vi "Browse for XNET Database.vi"(8 "error in (no error)":errorcluster) -> (0 "error out":errorcluster, 1 "Cancel Out":bool, 2 "Import Path out":path, 3 "XNET Settings":T1={"Database"="", "Cluster"="", "Port"="", "Baud rate [Bd]"=0, "Termination"=0, "CAN I/O Mode"=0, "FD Baud rate [Bd]"=500000, "Priority"=100, "Use Legacy"=FALSE, "FD ISO Mode"=0, "Default Max Counter Value"=0.0, "Default Protect Type"=enum."Arb ID + Bytes Checksum with Inversion"} {"FD ISO Mode" items=["ISO", "Non ISO", "ISO Legacy"]; "CAN I/O Mode" items=["CAN 2.0", "CAN FD", "CAN FD+BRS"]; "Termination" items=["Off", "On"]})   [LabVIEW 2025, in "Protection and Counter Addon System Explorer.lvlib"]
uses:
  Protection and Counter Addon System Explorer.lvlib
  Addon Shared/Types/XNET Settings.ctl
  SubModules/Frame-Protection-Support/Source/Shared/Types/Protection Type.ctl
  <resource>/objmgr/xnet.rc
  Addon Shared/Protection and Counter Addon Shared.lvlib
  SubModules/Frame-Protection-Support/Source/Shared/Protection and Counter Support Shared.lvlib
panel:
  in  "Path":path caption="Previous Personality Path (Optional)"
  in  "FD Baud rate [Bd]":u64=500000
  out "CAN I/O Mode":u32(ring) items=["CAN 2.0", "CAN FD", "CAN FD+BRS"]
  in  "Baud rate [Bd]":u64=500000
  in  "Select CAN Cluster":u16(ring)
  in  "Cancel":bool
  in  "Select":bool
  in  "XNET Database":refnum<k21>
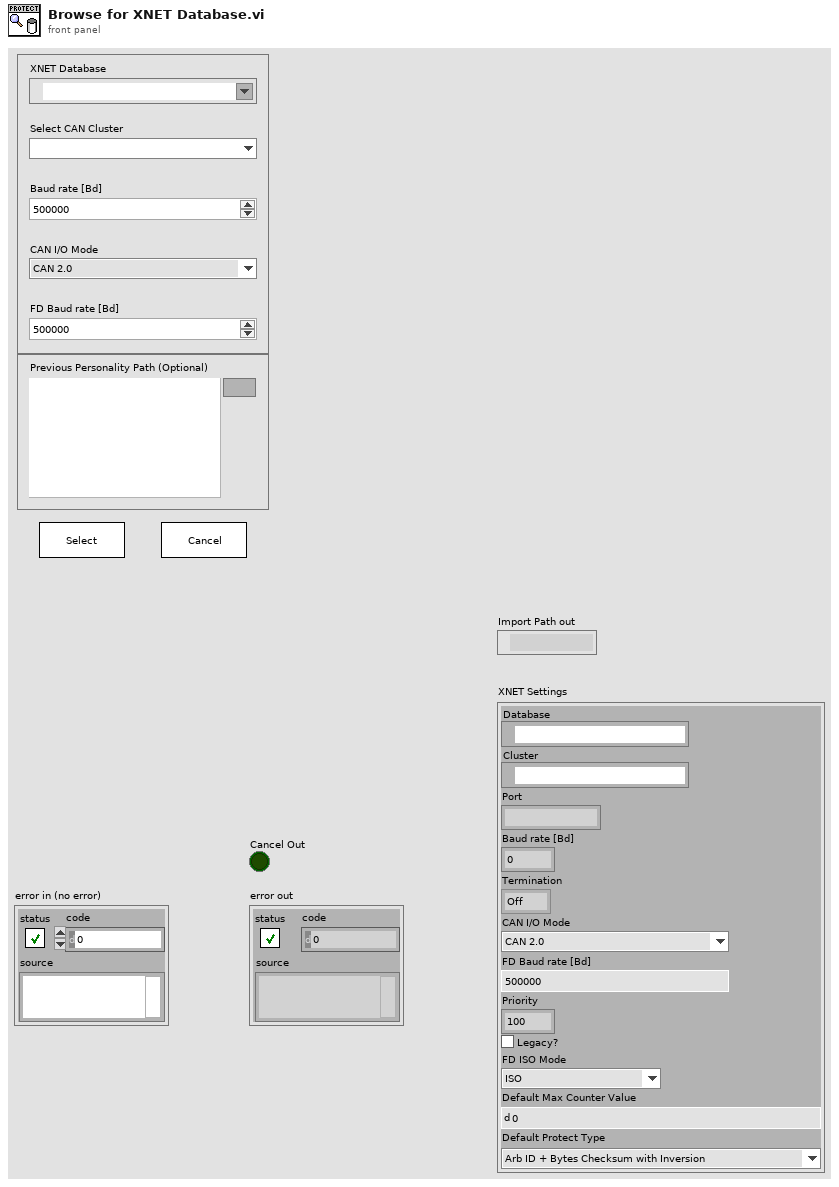
[diagram p1: front panel]
types:
  T1 = typedef "Protection and Counter Addon Shared.lvlib/XNET Settings.ctl" = cluster{"Database":refnum<k21>, "Cluster":refnum<k21>, "Port":string, "Baud rate [Bd]":u64, "Termination":u32, "CAN I/O Mode":u32, "FD Baud rate [Bd]":u64, "Priority":i32, "Use Legacy":bool, "FD ISO Mode":u32, "Default Max Counter Value":dbl, "Default Protect Type":T2}
  T2 = typedef "Protection and Counter Support Shared.lvlib/Protection Type.ctl" = enum16{"Arb ID + Bytes Checksum with Inversion", "Arb ID + Bytes CRC with Inversion", "Reversed Raw Signal Checksum with Inversion", "Concatenated Two's Compliment"}
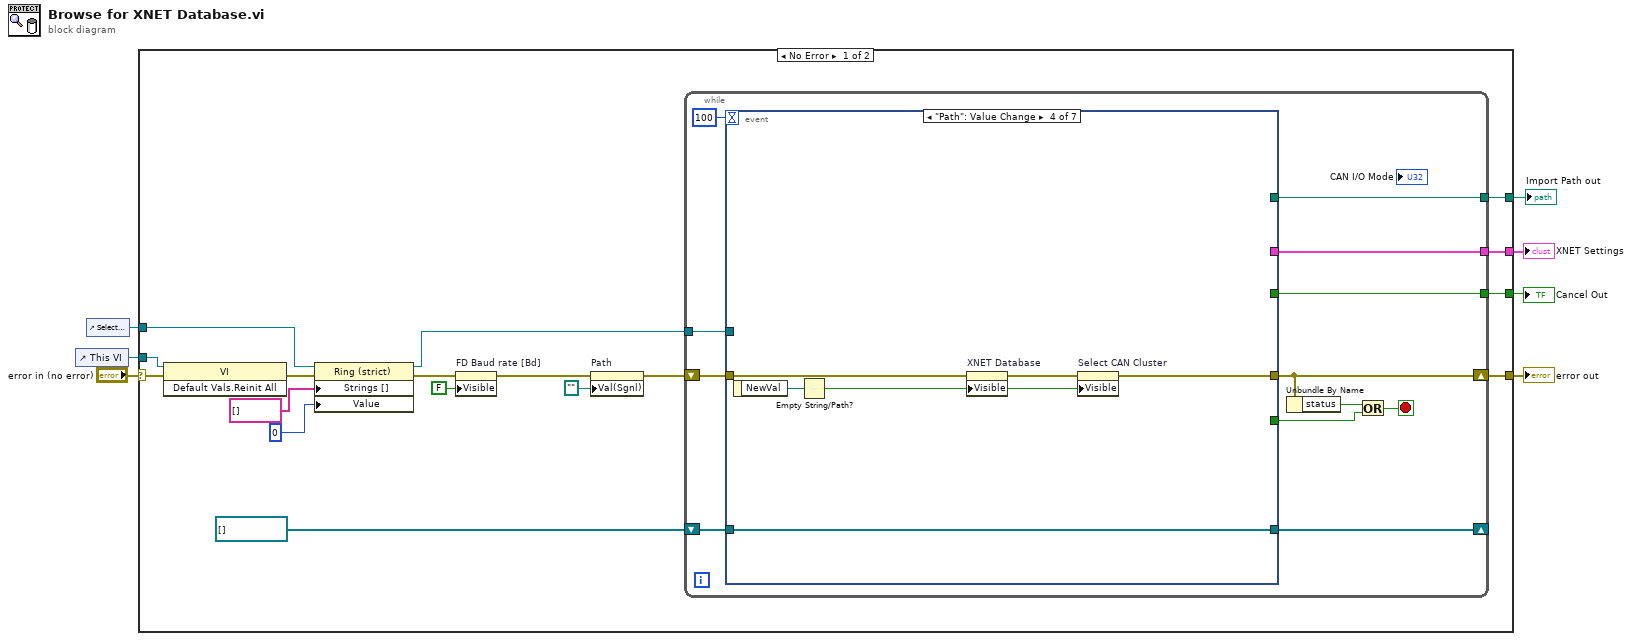
[diagram p0: block diagram]
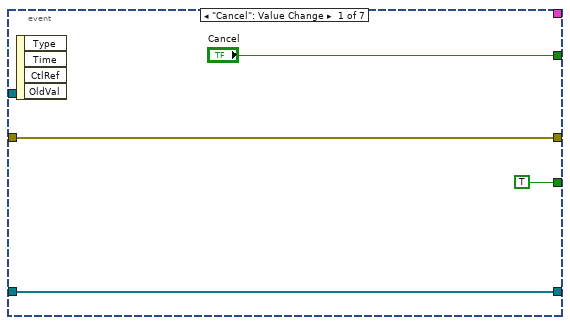
[diagram p2: hidden frame]
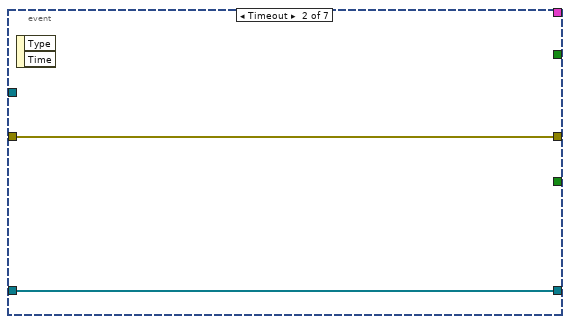
[diagram p3: hidden frame]
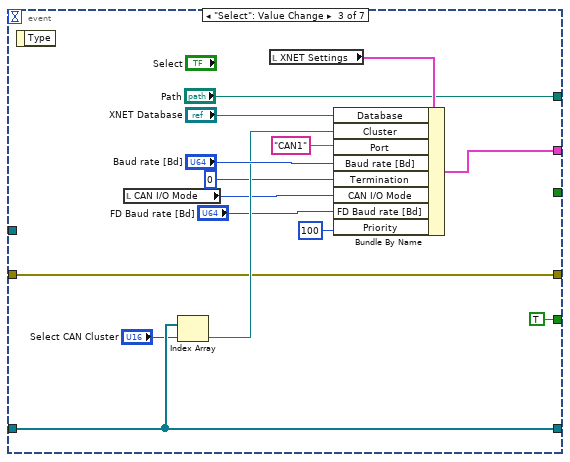
[diagram p4: hidden frame]
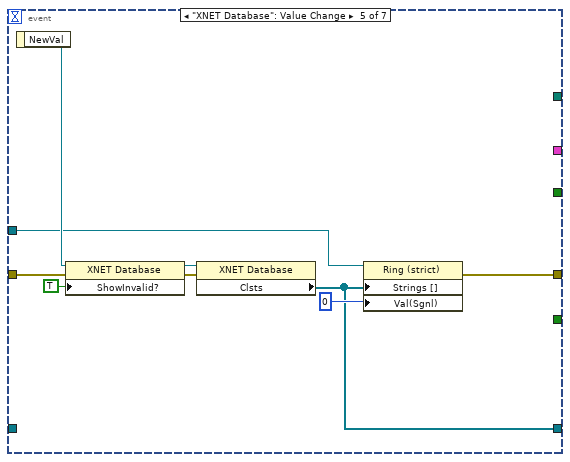
[diagram p5: hidden frame]
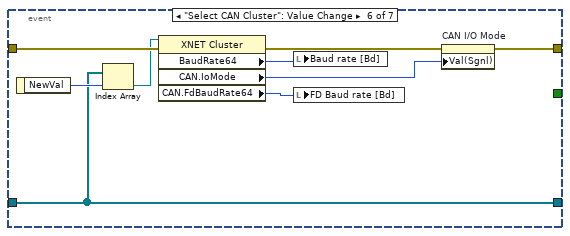
[diagram p6: hidden frame]
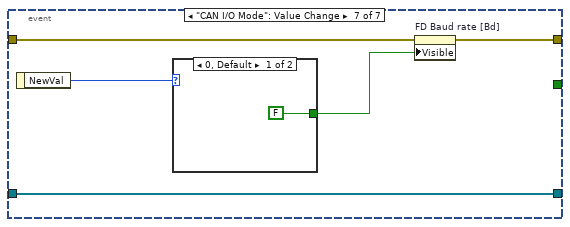
[diagram p7: hidden frame]
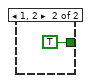
[diagram p8: hidden frame]
diagram:
  n1 = control-ref of="This VI"() -> (w4:refnum<vi>)
  n2 = control-ref of="Select CAN Cluster"() -> (w2:refnum<vi>)
  n3 = case shown="No Error" "error in (no error)" {
    selector: "error in (no error)" -> [w23 w89]
    tunnel: [w21 w89] -> w6
    tunnel: [w24 _] -> w5
    tunnel: w4 -> [w22 _]
    tunnel: [w19 _] -> w3
    tunnel: w2 -> [w18 _]
    tunnel: [w11 _] -> w1
    frame No Error {
      n4 = invoke class="VI" method="Default Vals.Reinit All"(reference=w22, error in=w23) -> (error out=w17:errorcluster)  [unwired: 1 in, 2 out]
      n5 = property on="Property Node" class="Ring (strict)"(reference=w18, error in=w17, "Strings []"=string[] [], "Value"=u16 0) -> (reference out=w16:refnum<vi>, error out=w13:errorcluster)
      n6 = property on="FD Baud rate [Bd]" class="DigNum (strict)"(error in=w13, "Visible"=FALSE) -> (error out=w10:errorcluster)  [unwired: 1 in, 1 out]
      n7 = property on="Path" class="Path"(error in=w10, "Val(Sgnl)"=path "") -> (error out=w9:errorcluster)  [unwired: 1 in, 1 out]
      n8 = while {
        tunnel: [w36] -> w24
        shift-right: [w34] -> _
        shift-left: refnum<k21>[] [] ("Clsts") -> [w33]
        shift-right: [w30] -> w21
        shift-left: w9 -> [w35]
        tunnel: [w32] -> w19
        tunnel: w16 -> [w26]
        tunnel: [w25] -> w11
        stop <- w27 stop-if-true
        n9 = event shown="[3] \"Path\": Value Change" {
          selector: _ -> [_ _ _ _ _ _ _]
          dyn-events: _ -> [_ _ _ _ _ _ _]
          timeout: 100 -> [_ _ _ _ _ _ _]
          tunnel: ["Cancel" _ _ _ _ _ _] -> w36
          tunnel: w35 -> [w38 w42 w49 w58 w69 w80 w86]
          tunnel: [w39 w41 w54 w63 w66 w77 w84] -> w34
          tunnel: w33 -> [w39 w41 w54 w63 _ w77 w84]
          tunnel: [w38 w42 w49 w59 w64 w75 w85] -> w30
          tunnel: [_ _ w51 _ _ _ _] -> w32
          tunnel: [TRUE _ TRUE _ _ _ _] -> w28
          tunnel: w26 -> [_ _ _ _ w65 _ _]
          tunnel: [_ _ "Path" _ _ _ _] -> w25
          event "Cancel": Value Change {
            n10 = event-data() -> ()  [unwired: 1 in, 4 out]
          }
          event Timeout {
            n11 = event-data() -> ()  [unwired: 1 in, 2 out]
          }
          event "Select": Value Change {
            n12 = event-data() -> ()  [unwired: 1 in, 1 out]
            n13 = local read "CAN I/O Mode"() -> (w44:u32)
            n14 = Index Array(array=w54, index="Select CAN Cluster") -> (element=w52:refnum<k21>)
            n15 = local read "XNET Settings"() -> (w55:T1)
            n16 = Bundle By Name(cluster=w55, "Database"="XNET Database", "Cluster"=w52, "Port"="CAN1", "Baud rate [Bd]"="Baud rate [Bd]", "Termination"=u32 0, "CAN I/O Mode"=w44, "FD Baud rate [Bd]"="FD Baud rate [Bd]", "Priority"=100) -> (w51:T1)
          }
          event "Path": Value Change {
            n17 = event-data() -> ("NewVal"=w62:path)  [unwired: 1 in]
            n18 = Empty String/Path?(string/path=w62) -> (empty?=w61:bool)
            n19 = property on="XNET Database" class="XNET (strict)"(error in=w58, "Visible"=w61) -> (error out=w60:errorcluster)  [unwired: 1 in, 1 out]
            n20 = property on="Select CAN Cluster" class="Ring (strict)"(error in=w60, "Visible"=w61) -> (error out=w59:errorcluster)  [unwired: 1 in, 1 out]
          }
          event "XNET Database": Value Change {
            n21 = event-data() -> ("NewVal"=w68:refnum<k21>)  [unwired: 1 in]
            n22 = property class="XNET Database"(reference=w68, error in=w69, "ShowInvalid?"=TRUE ("Show Invalid From Open?")) -> (reference out=w72:refnum<k21>, error out=w71:errorcluster)
            n23 = property class="XNET Database"(reference=w72, error in=w71) -> ("Clsts"=w66:refnum<k21>[])  [unwired: 2 out]
            n24 = property on="Property Node" class="Ring (strict)"(reference=w65, "Strings []"=w66, "Val(Sgnl)"=u16 0 ("Value (Signaling)")) -> (error out=w64:errorcluster)  [unwired: 1 in, 1 out]
          }
          event "Select CAN Cluster": Value Change {
            n25 = event-data() -> ("NewVal"=w79:u16)  [unwired: 1 in]
            n26 = Index Array(array=w77, index=w79) -> (element=w78:refnum<k21>)
            n27 = property class="XNET Cluster"(reference=w78, error in=w80) -> (error out=w74:errorcluster, "BaudRate64"=w81:u64, "CAN.IoMode"=w73:u32, "CAN.FdBaudRate64"=w76:u64)  [unwired: 1 out]
            n28 = local write "Baud rate [Bd]"(w81) -> ()
            n29 = local write "FD Baud rate [Bd]"(w76) -> ()
            n30 = property on="CAN I/O Mode" class="Ring (strict)"(error in=w74, "Val(Sgnl)"=w73) -> (error out=w75:errorcluster)  [unwired: 1 in, 1 out]
          }
          event "CAN I/O Mode": Value Change {
            n31 = event-data() -> ("NewVal"=w82:u32)  [unwired: 1 in]
            n32 = case shown="0, Default" w82 {
              tunnel: [FALSE TRUE] -> w83
              frame 0, Default {
              }
              frame 1, 2 {
              }
            }
            n33 = property on="FD Baud rate [Bd]" class="DigNum (strict)"(error in=w86, "Visible"=w83) -> (error out=w85:errorcluster)  [unwired: 1 in, 1 out]
          }
        }
        n34 = Unbundle By Name(w30) -> ("status"=w29:bool)
        n35 = Or(x=w29, y=w28) -> (x .or. y?=w27:bool)
      }
    }
    frame Error {
    }
  }
  "error out" <- w6
  "Cancel Out" <- w5
  "XNET Settings" <- w3
  "Import Path out" <- w1
